vi "Wait For MV Flag.vi"(6 "WaitMode(T=Stop)":bool, 7 "Timeout(0.5S Cycles)":i32, 8 "error in (no error)":errorcluster, 9 "Device Name":string, 10 "Mdrive Mode":T1, 11 "VISA Refnum in":refnum<visa-resource-name>) -> (0 "error out":errorcluster, 2 "OK":bool, 3 "VISA Refnum out":refnum<visa-resource-name>)   [LabVIEW 2015]
uses:
  MCode_LV_86/MDrive Mode.ctl
  MCode_LV_86/Get Parameter.ctl
  Stream/LP Globals.vi
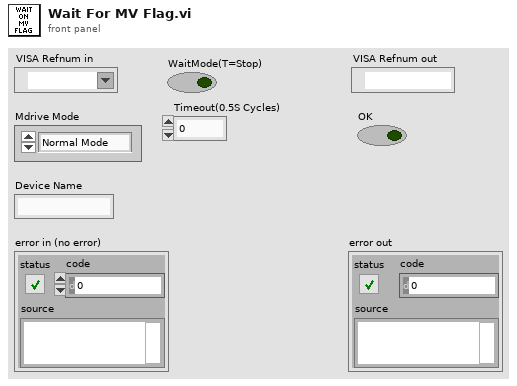
[diagram p1: front panel]
types:
  T1 = typedef "MDrive Mode.ctl" = enum16{"Normal Mode", "Party Mode"}
  T2 = typedef "Get Parameter.ctl" = enum16{"Acceleration (A)", "Baud Rate (BD)", "Busy Flag (BY)", "Counter 1 (C1)", "Counter 2 (C2)", "Check Sum Enable (CK)", "Clock Mode (CM)", "Clock Mode Ratio (CR)", "Clock Mode Out Step Width (CW)", "Deceleration (D)", "Digital Filtering, Input 1 (D1)", "Digital Filtering, Input 2 (D2)", "Digital Filtering, Input 3 (D3)", "Digital Filtering, Input 4 (D4)", "Digital Filtering, Input 5 (D5)", "Digital Filtering, Input 9 (D9)", "Digital Filtering, Input 10 (D10)", "Digital Filtering, Input 11 (D11)", "Digital Filtering, Input 12 (D12)", "Deadband (DB)", "Enable/Disable Drive (DE)", "Device Name (DN)", "End Program Execution (E)", "Encoder Function Enable (EE)", "Encoder Lines (EL)", "Error Flag (EF)", "Error Variable (ER)", "Echo Mode (EM)", "Escape (ES)", "Execute Program at Address (EX)", "Hold Current (HC)", "Hold Current Delay Time (HI)", "Input 1 (I1)", "Input 2 (I2)", "Input 3 (I3)", "Input 4 (I4)", "Input 5 Analog (I5)", "Input 6 Encoder Index (I6)", "Input 9 (I9)", "Input 10 (I10)", "Input 11 (I11)", "Input 12 (I12)", "Input Low Byte (1-4) (IL)", "Input High Byte (9-12) (IH)", "Inputs Total (1-4,9-12) (IN)", "Internal Temperature (IT)", "Jog Enable (JE)", "Limit Stop Mode (LM)", "MicroStepping Select (MS)", "Motor Settling Delay Time (MT)", "Moving Flag (MV)", "Output 1 (O1)", "Output 2 (O2)", "Output 3 (O3)", "Output 4 (O4)", "Output 9 (O9)", "Output 10 (O10)", "Output 11 (O11)", "Output 12 (O12)", "Output High Byte (9-12) (OH)", "Output Low Byte (1-4) (OL)", "Output Total (1-4 and 9-12) (OT)", "Position (P)", "Position Captured at Trip (PC)", "Position Maintenance (PM)", "Part Number (PN)", "Party Mode (PY)", "Register 1 (R1)", "Register 2 (R2)", "Register 3 (R3)", "Register 4 (R4)", "Run Current (RC)", "Serial Number (SN)", "Stall Flag (ST)", "Stall Factor (SF)", "Stall Mode Set (SM)", "User Variables (UV)", "Velocity (V)", "Velocity Changing Flag (VC)", "Velocity Initial (VI)", "Version, Firmware (VR)", "Velocity Maximum (VM)", "Read Input1", "Read Input2"}
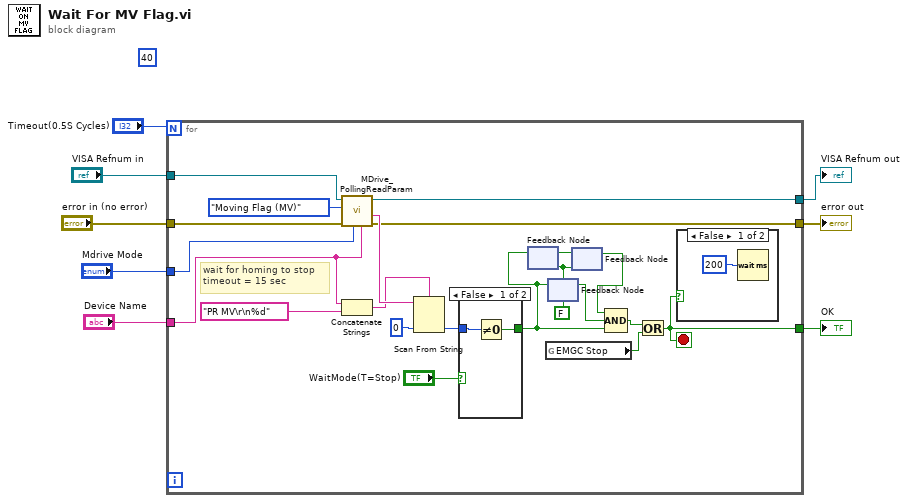
[diagram p0: block diagram]
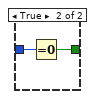
[diagram p2: hidden frame]
diagram:
  (unwired) 40
  n1 = for {
    N: "Timeout(0.5S Cycles)" -> [_]
    tunnel: "VISA Refnum in" -> [w23]
    tunnel: "error in (no error)" -> [w22]
    tunnel: [w21] -> w5
    tunnel: [w20] -> w4
    tunnel: "Device Name" -> [w18]
    tunnel: "Mdrive Mode" -> [w19]
    tunnel: [w17] -> w3
    stop <- w17 stop-if-true
    w9 = FALSE
    # "wait for homing to stop\ntimeout = 15 sec"
    n2 = call "MDrive_PollingReadParam.vi"("Device Name"=w18, "Mdrive Mode"=w19, "error in (no error)"=w22, "Get Parameter"=Get_Parameter."Moving Flag (MV)", "VISA Refnum in"=w23) -> ("error out"=w21:errorcluster, "String"=w28:string, "VISA Refnum out"=w20:refnum<visa-resource-name>)  [unwired: 3 in, 1 out]
    n3 = Concatenate Strings(w18, "PR MV\r\n%d" ("format string")) -> (w26:string)
    n4 = Scan From String(format string=w26, input string=w28, default 1=0 ("output 1")) -> (output 1=w29:i32)  [unwired: 2 in, 3 out]
    n5 = case shown="False" "WaitMode(T=Stop)" {
      tunnel: w29 -> [w31 w33]
      tunnel: [w30 w32] -> w12
      frame False {
        n6 = Not Equal To 0?(x=w31) -> (x != 0?=w30:bool)
      }
      frame True {
        n7 = Equal To 0?(x=w33) -> (x = 0?=w32:bool)
      }
    }
    n8 = feedback #1(w9) -> (w11:bool)
    n9 = feedback-in #1(w12) -> ()
    n10 = global read "LP Globals.vi" "EMGC Stop"() -> (w16:bool)
    n11 = feedback-in #2(w12) -> ()
    n12 = feedback #2(w9) -> (w15:bool)
    n13 = feedback #3(w9) -> (w10:bool)
    n14 = feedback-in #3(w11) -> ()
    n15 = Compound Arithmetic op=AND(w10, w15, w12) -> (w14:bool)
    n16 = Or(x=w14, y=w16) -> (x .or. y?=w17:bool)
    n17 = case shown="False" w17 {
      frame False {
        n18 = Wait (ms)(milliseconds to wait=u32 200) -> ()  [unwired: 1 out]
      }
      frame True {
      }
    }
  }
  "error out" <- w5
  "VISA Refnum out" <- w4
  "OK" <- w3
